vi "Update Sample Meta Data.vi"(8 "error in":errorcluster, 10 "Item Info":T1, 11 "MetaDataObj":refnum<class "MetaDataObj.lvclass">) -> (0 "error out":errorcluster, 3 "MetaDataObj out":refnum<class "MetaDataObj.lvclass">)   [LabVIEW 2021]
uses:
  <resource>/dialog/NewProjectWizard/MetaDataObj/MetaDataObj.lvclass
  Control/Item Info.ctl
  <resource>/dialog/NewProjectWizard/MetaDataObj/Accessors/Read Project Path.vi
  <resource>/dialog/NewProjectWizard/MetaDataObj/Accessors/Write Project Path.vi
  <resource>/dialog/NewProjectWizard/MetaDataObj/Accessors/Write LocationPath.vi
  <resource>/dialog/NewProjectWizard/MetaDataObj/Accessors/Write Description.vi
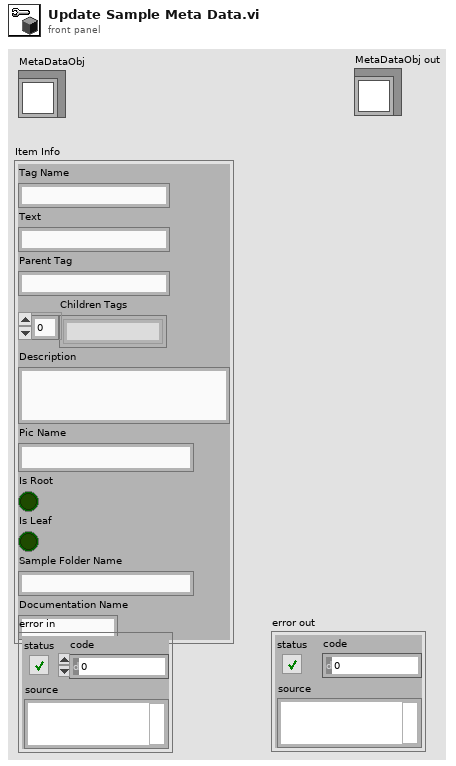
[diagram p1: front panel]
types:
  T1 = typedef "Item Info.ctl" = cluster{"Tag Name":string, "Text":string, "Parent Tag":string, "Children Tags":string[], "Description":string, "Pic Name":string, "Is Root":bool, "Is Leaf":bool, "Sample Folder Name":string, "Documentation Name":string}
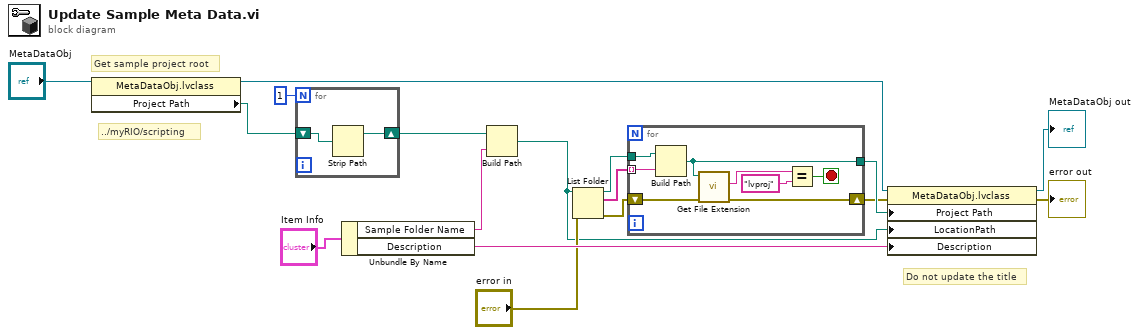
[diagram p0: block diagram]
diagram:
  # "../myRIO/scripting"
  # "Do not update the title"
  # "Get sample project root"
  n1 = property class="MetaDataObj.lvclass"(reference="MetaDataObj") -> (reference out=w16:refnum<class "MetaDataObj.lvclass">, "Project Path"=w14:path)  [unwired: 1 in, 1 out]
  n2 = for {
    N: 1 -> [_]
    shift-right: [w18] -> w13
    shift-left: w14 -> [w19]
    n3 = Strip Path(path=w19) -> (stripped path=w18:path)  [unwired: 1 out]
  }
  n4 = Unbundle By Name("Item Info") -> ("Sample Folder Name"=w12:string, "Description"=w7:string)
  n5 = Build Path(base path=w13, name or relative path=w12) -> (appended path=w1:path)
  n6 = List Folder(path=w1, error in="error in") -> (path out=w10:path, filenames=w11:string[], error out=w9:errorcluster)  [unwired: 2 in, 1 out]
  n7 = for {
    tunnel: w11 -> [w26] mode=indexing
    tunnel: w10 -> [w27]
    shift-right: [w20] -> w5
    shift-left: w9 -> [w25]
    tunnel: [w21] -> w8
    stop <- w22 stop-if-true
    n8 = Build Path(base path=w27, name or relative path=w26) -> (appended path=w21:path)
    n9 = call <vilib>:"Get File Extension.vi"("error in (no error)"=w25, "file"=w21) -> ("error out"=w20:errorcluster, "lowercase file extension"=w24:string)  [unwired: 5 in, 3 out]
    n10 = Equal?(x=w24, y="lvproj") -> (x = y?=w22:bool)
  }
  n11 = property class="MetaDataObj.lvclass"(reference=w16, error in=w5, "Project Path"=w8, "LocationPath"=w1, "Description"=w7) -> (reference out=→"MetaDataObj out":refnum<class "MetaDataObj.lvclass">, error out=→"error out":errorcluster)
